vi "ai_oneshot_full.vi"() -> ()   [LabVIEW 2020]
uses:
  <vilib>/Analysis/baseanly.llb/Mean (DBL).vi
  <vilib>/Analysis/NI_AALBase.lvlib
panel:
  out "数组":dbl[](array[numeric]) format="%_6g"
  in  "AiOneShotPoints":u32=1000
  out "error out":errorcluster caption="错误输出"
  out "AiFifoResidual":i32
  out "波形图":sgl[][](graph)
  in  "SamplePeriod(ns)":u32=5000
  in  "ChanSel":bool[](array[boolean])=[TRUE, TRUE, TRUE, TRUE, TRUE, TRUE, TRUE, TRUE, FALSE, FALSE, FALSE, FALSE, FALSE, FALSE, FALSE, FALSE, FALSE, FALSE, FALSE, FALSE, FALSE, FALSE, FALSE, FALSE]
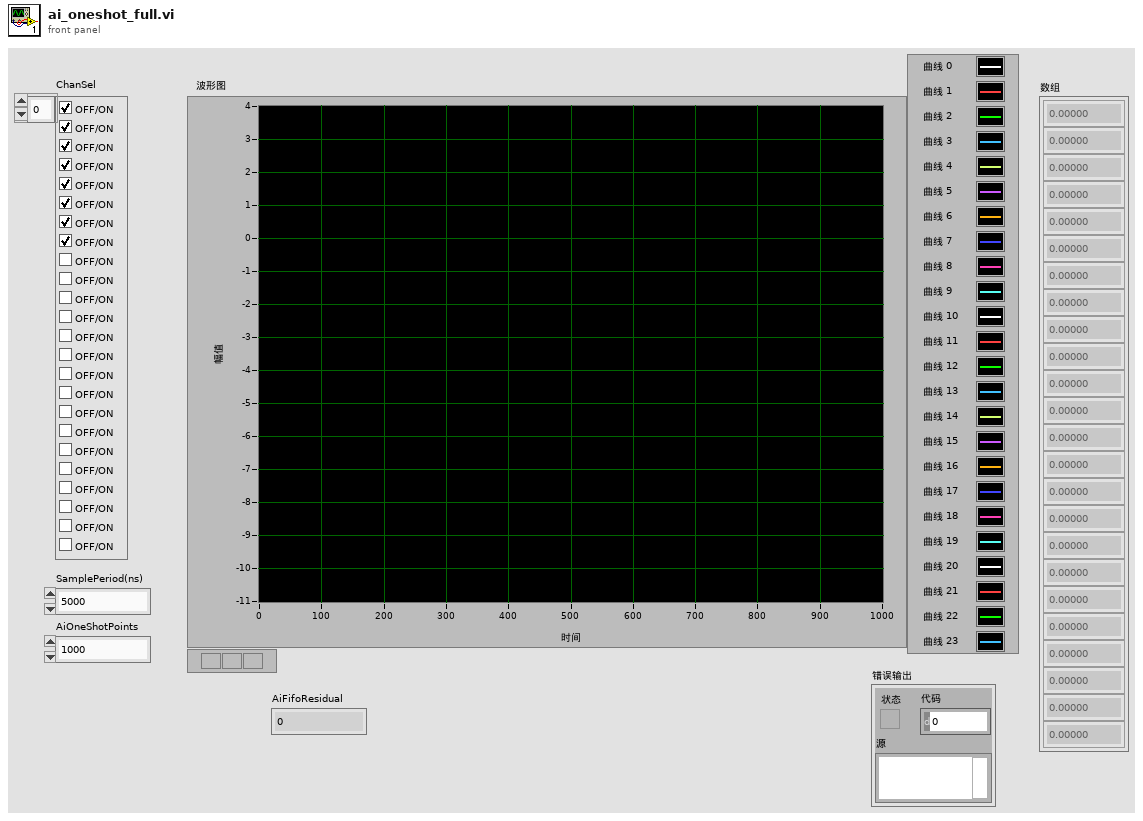
[diagram p1: front panel]
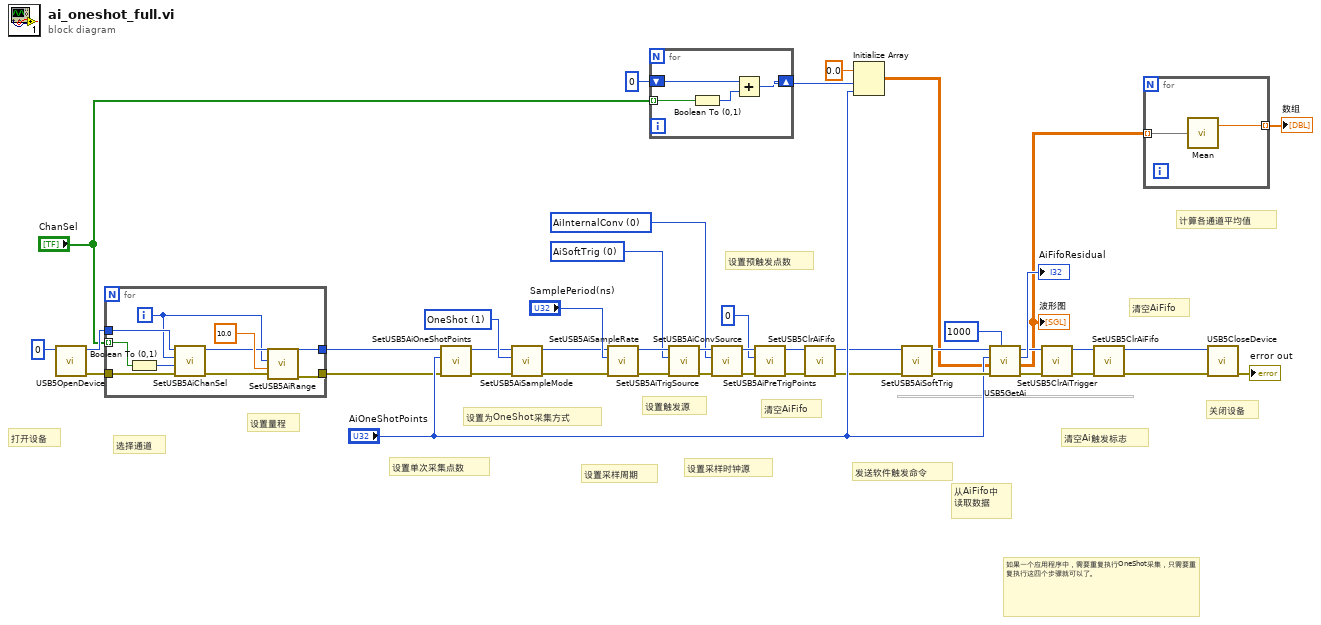
[diagram p0: block diagram]
diagram:
  w2 = u8 0 items=["AiInternalConv"=0, "ConvIn"=1, "DiConv"=3, "DoConv"=4, "Ao0Conv"=5, "Ao1Conv"=6, "Ao2Conv"=7, "Ao3Conv"=8] ("AiConvSource")
  w3 = u8 0 items=["AiSoftTrig"=0, "ExtTrigIn"=1, "Din0RisingEdge"=2, "Din1RisingEdge"=3, "Din2RisingEdge"=4, "Din3RisingEdge"=5, "WithDiTrig"=7, "WithDoTrig"=8, "WithAo0Trig"=9, "WithAo1Trig"=10, "WithAo2Trig"=11, "WithAo3Trig"=12, "GlobalSoftTrig"=255] ("AiTrigSource")
  w40 = u8 1 items=["Continuous", "OneShot"] ("AiSampleMode")
  # "设置量程"
  # "如果一个应用程序中，需要重复执行OneShot采集，只需要重复执行这四个步骤就可以了。"
  # "计算各通道平均值"
  # "关闭设备"
  # "清空AiFifo"
  # "清空Ai触发标志"
  # "从AiFifo中\n读取数据"
  # "发送软件触发命令"
  # "清空AiFifo"
  # "设置预触发点数"
  # "设置采样时钟源"
  # "设置触发源"
  # "设置采样周期"
  # "设置为OneShot采集方式"
  # "设置单次采集点数"
  # "选择通道"
  # "打开设备"
  n1 = call "USB5OpenDevice.vi"("DevIndex"=0) -> ("error out"=w41:errorcluster, "DevIndex Out"=w42:i32)  [unwired: 9 in]
  n2 = for {
    tunnel: w42 -> [w53]
    tunnel: w41 -> [w52]
    tunnel: [w45] -> w5
    tunnel: [w44] -> w4
    tunnel: "ChanSel" -> [w50] mode=indexing
    i -> [w47]
    n3 = Boolean To (0,1)(Boolean=w50) -> (0, 1=w51:i16)
    n4 = call "SetUSB5AiChanSel.vi"("错误输入（无错误）"=w52, "Sel"=w51, "Chan"=w47, "DevIndex"=w53) -> ("错误输出"=w46:errorcluster, "DevIndex Out"=w48:i32)  [unwired: 6 in]
    n5 = call "SetUSB5AiRange.vi"("错误输入（无错误）"=w46, "AiRange"=sgl 10.0, "Chan"=w47, "DevIndex"=w48) -> ("错误输出"=w44:errorcluster, "DevIndex Out"=w45:i32)  [unwired: 6 in]
  }
  n6 = call "SetUSB5AiOneShotPoints.vi"("错误输入（无错误）"=w4, "AiOneShotPoints"="AiOneShotPoints", "DevIndex"=w5) -> ("错误输出"=w27:errorcluster, "DevIndex Out"=w28:i32)  [unwired: 7 in]
  n7 = call "SetUSB5AiSampleMode.vi"("错误输入（无错误）"=w27, "AiSampleMode"=w40, "DevIndex"=w28) -> ("错误输出"=w6:errorcluster, "DevIndex Out"=w7:i32)  [unwired: 7 in]
  n8 = call "SetUSB5AiSampleRate.vi"("错误输入（无错误）"=w6, "SamplePeriod(ns)"="SamplePeriod(ns)", "DevIndex"=w7) -> ("错误输出"=w15:errorcluster, "DevIndex Out"=w16:i32)  [unwired: 7 in]
  n9 = for {
    tunnel: "ChanSel" -> [w57] mode=indexing
    shift-right: [w54] -> w31
    shift-left: i16 0 -> [w55]
    n10 = Boolean To (0,1)(Boolean=w57) -> (0, 1=w56:i16)
    n11 = Add(x=w55, y=w56) -> (x+y=w54:i16)
  }
  n12 = call "SetUSB5AiTrigSource.vi"("错误输入（无错误）"=w15, "AiTrigSource"=w3, "DevIndex"=w16) -> ("错误输出"=w18:errorcluster, "DevIndex Out"=w17:i32)  [unwired: 7 in]
  n13 = call "SetUSB5AiConvSource.vi"("错误输入（无错误）"=w18, "AiConvSource"=w2, "DevIndex"=w17) -> ("错误输出"=w20:errorcluster, "DevIndex Out"=w19:i32)  [unwired: 7 in]
  n14 = call "SetUSB5AiPreTrigPoints.vi"("错误输入（无错误）"=w20, "AiPreTrigPoints"=u32 0, "DevIndex"=w19) -> ("错误输出"=w13:errorcluster, "DevIndex Out"=w14:i32)  [unwired: 7 in]
  n15 = call "SetUSB5ClrAiFifo.vi"("错误输入（无错误）"=w13, "DevIndex"=w14) -> ("错误输出"=w12:errorcluster, "DevIndex Out"=w11:i32)  [unwired: 8 in]
  n16 = Initialize Array(sgl 0.0 ("元素"), w31, "AiOneShotPoints") -> (w10:sgl[][])
  n17 = call "SetUSB5AiSoftTrig.vi"("错误输入（无错误）"=w12, "DevIndex"=w11) -> ("错误输出"=w38:errorcluster, "DevIndex Out"=w39:i32)  [unwired: 8 in]
  n18 = call "USB5GetAi.vi"("TimeOut"=1000, "错误输入（无错误）"=w38, "Ai"=w10, "Points"="AiOneShotPoints", "DevIndex"=w39) -> ("错误输出"=w23:errorcluster, "Ai Out"=w8:sgl[][], "AiFifoUsed"=→"AiFifoResidual":i32, "DevIndex Out"=w24:i32)  [unwired: 3 in]
  "波形图" <- w8
  n19 = call "SetUSB5ClrAiTrigger.vi"("错误输入（无错误）"=w23, "DevIndex"=w24) -> ("错误输出"=w22:errorcluster, "DevIndex Out"=w25:i32)  [unwired: 8 in]
  n20 = call "SetUSB5ClrAiFifo.vi"("错误输入（无错误）"=w22, "DevIndex"=w25) -> ("错误输出"=w34:errorcluster, "DevIndex Out"=w33:i32)  [unwired: 8 in]
  n21 = for {
    tunnel: w8 -> [w59] mode=indexing
    tunnel: [w58] -> w9 mode=indexing
    n22 = call-poly <vilib>:"Mean.vi"("X"=w59) -> ("mean"=w58:dbl)  [unwired: 1 out]
  }
  "数组" <- w9
  n23 = call "USB5CloseDevice.vi"("错误输入（无错误）"=w34, "DevIndex"=w33) -> ("error out"=→"error out":errorcluster)  [unwired: 8 in, 1 out]
